vi "32to64bitTimestamp.vi"(1 "Timestamp bitness":string(combo)="32", 2 "Timestamps In":u64[](array[numeric])=[10, 20, 30, 5, 15, 25, 5, 15]) -> (0 "Timestamps Out":u64[](array[numeric]))   [LabVIEW 2014]
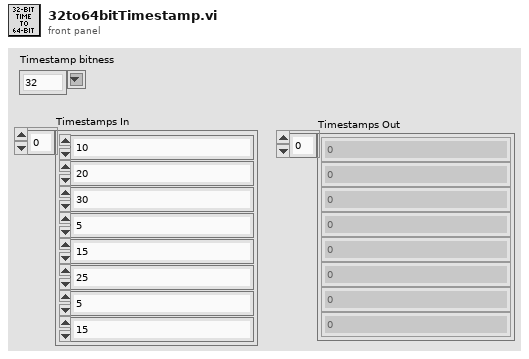
[diagram p1: front panel]
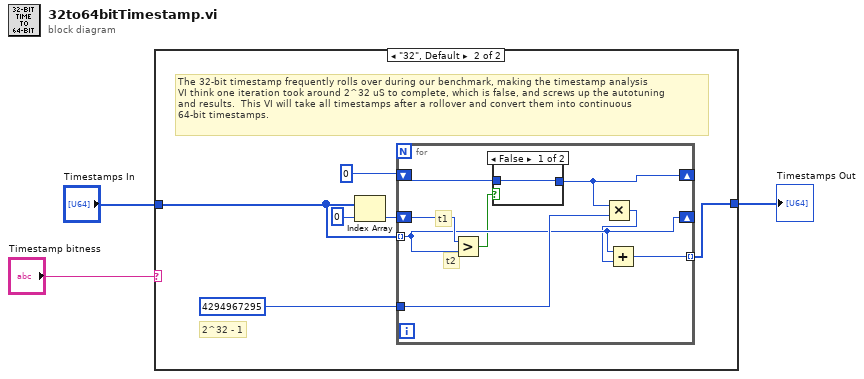
[diagram p0: block diagram]
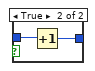
[diagram p3: hidden frame]
diagram:
  n1 = case shown="\"32\", Default" "Timestamp bitness" {
    tunnel: "Timestamps In" -> [w4 w10]
    tunnel: [w4 w5] -> w1
    frame "64" {
      # "If the timestamp has 64-bit precision, we're not going to do the adjustment (assume\nthe chances are too low that we'll roll over the u64)."
    }
    frame "32", Default {
      # "The 32-bit timestamp frequently rolls over during our benchmark, making the timestamp analysis\nVI think one iteration took around 2^32 uS to complete, which is false, and screws up the autotuning\nand results.  This VI will take all timestamps after a rollover and convert them into continuous\n64-bit timestamps."
      # "2^32 - 1"
      n2 = Index Array(array=w10, index=0) -> (element=w8:u64)
      n3 = for {
        tunnel: w10 -> [w13] mode=indexing
        shift-right: [w13] -> _
        shift-left: w8 -> [w17]
        tunnel: u64 4294967295 -> [w18]
        tunnel: [w16] -> w5 mode=indexing
        shift-right: [w14] -> _
        shift-left: 0 -> [w15]
        # "t1"
        # "t2"
        n4 = Greater?(x=w17, y=w13) -> (0:w11:bool)
        n5 = case shown="False" w11 {
          tunnel: w15 -> [w19 w21]
          tunnel: [w19 w20] -> w14
          frame False {
          }
          frame True {
            n6 = Increment(x=w21) -> (x+1=w20:i32)
          }
        }
        n7 = Multiply(x=w14, y=w18) -> (x*y=w12:u64)
        n8 = Add(x=w13, y=w12) -> (x+y=w16:u64)
      }
    }
  }
  "Timestamps Out" <- w1
